vi "TP1.2.vi"() -> ()   [LabVIEW 2013]
panel:
  in  "Boolean":bool
  out "Waveform Graph":dbl[](graph)
  in  "Cantidad de Muestras":i32=1000
  in  "Amplitud":dbl=10.0
  in  "Frecuencia":dbl=5.0
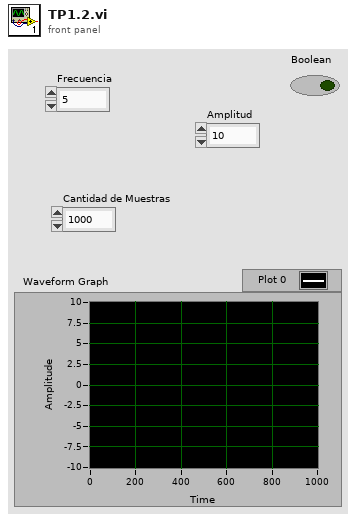
[diagram p1: front panel]
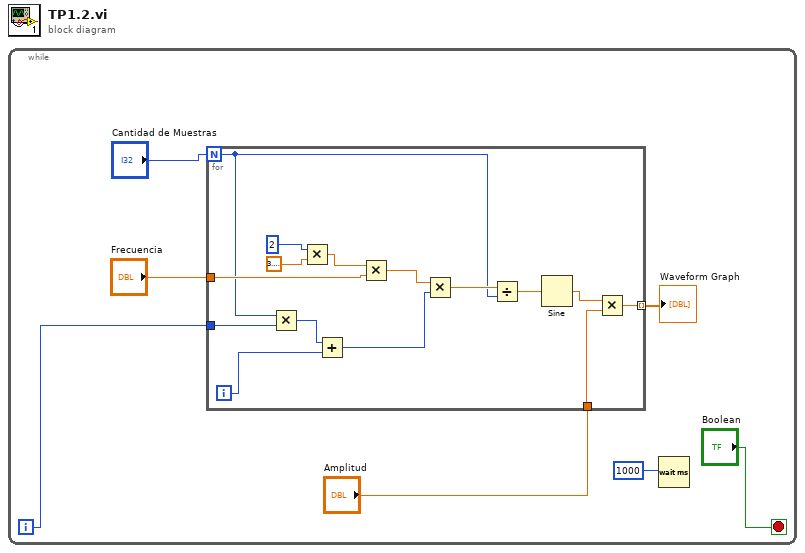
[diagram p0: block diagram]
diagram:
  n1 = while {
    i -> [w3]
    stop <- "Boolean" stop-if-true
    n2 = for {
      N: "Cantidad de Muestras" -> [w11]
      tunnel: "Frecuencia" -> [w16]
      tunnel: "Amplitud" -> [w15]
      tunnel: [w13] -> w5 mode=indexing
      tunnel: w3 -> [w10]
      i -> [w12]
      n3 = Multiply(x=w11, y=w10) -> (x*y=w9:i32)
      n4 = Multiply(x=2, y=3.141592653589793) -> (x*y=w20:dbl)
      n5 = Add(x=w9, y=w12) -> (x+y=w8:i32)
      n6 = Multiply(x=w20, y=w16) -> (x*y=w19:dbl)
      n7 = Multiply(x=w19, y=w8) -> (x*y=w18:dbl)
      n8 = Divide(x=w18, y=w11) -> (x/y=w17:dbl)
      n9 = Sine(x=w17) -> (sin(x)=w14:dbl)
      n10 = Multiply(x=w14, y=w15) -> (x*y=w13:dbl)
    }
    "Waveform Graph" <- w5
    n11 = Wait (ms)(milliseconds to wait=1000) -> ()  [unwired: 1 out]
  }
